vi "Main (RT).vi"() -> ()   [LabVIEW 2015]
uses:
  BMP085 (GY-65) Library/BMP085 (RT).lvlib
panel:
  out "History":cluster{"Temp [°C]":dbl, "hPa":dbl}(graph)
  in  "Stop Button":bool
  out "Pressure [hPa]":dbl(knob) scale=900.0..1100.0
  out "Temperature [°C]":dbl(slide) scale=0.0..80.0
  # "952"
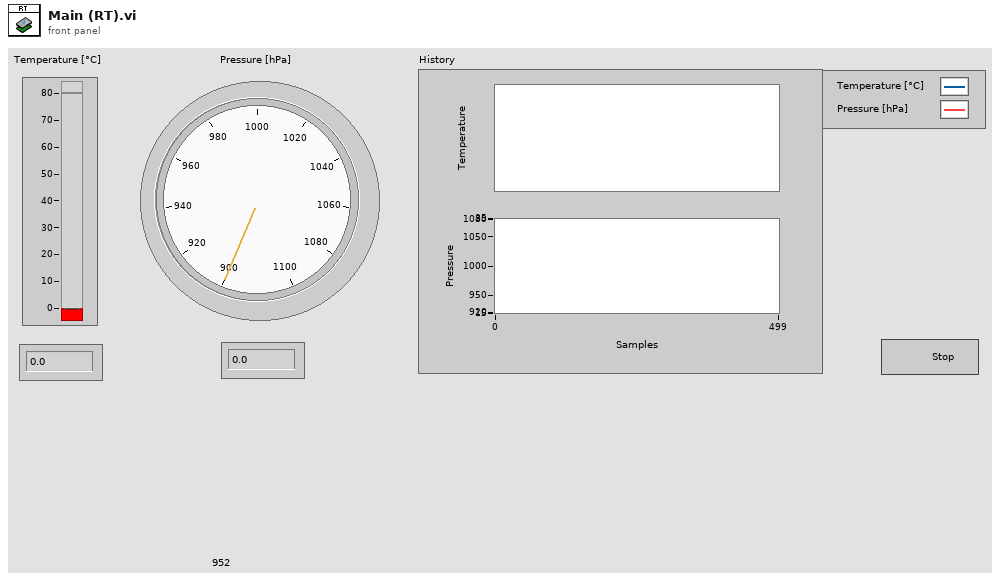
[diagram p1: front panel]
types:
  T1 = enum8{"ultra low power", "standard", "high resolution", "ultra high resolution"}
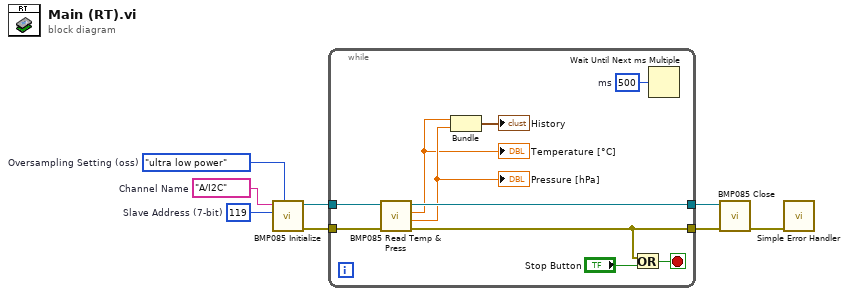
[diagram p0: block diagram]
diagram:
  w3 = u8 119  # Slave Address (7-bit)
  w4 = T1."ultra low power"  # Oversampling Setting (oss)
  w5 = tag "A/I2C"  # Channel Name
  n1 = call "BMP085 Initialize.vi"("Oversampling Setting (oss)"=w4, "Slave Address (7-bit)"=w3, "Channel Name"=w5) -> ("error out"=w7:errorcluster, "BMP085 (GY-65) out"=w8:refnum<class "BMP085 (GY-65).lvclass">)  [unwired: 7 in]
  n2 = while {
    tunnel: w8 -> [w18]
    tunnel: [w17] -> w1
    tunnel: w7 -> [w16]
    tunnel: [w14] -> w6
    stop <- w15 stop-if-true
    w12 = u32 500  # ms
    # "Example: BMP085"
    n3 = call "BMP085 Read Temp & Press.vi"("error in (no error)"=w16, "BMP085 (GY-65) in"=w18) -> ("error out"=w14:errorcluster, "hPa"=w11:dbl, "Temp [°C]"=w10:dbl, "BMP085 (GY-65) out"=w17:refnum<class "BMP085 (GY-65).lvclass">)  [unwired: 6 in]
    "Pressure [hPa]" <- w11
    "Temperature [°C]" <- w10
    n4 = Bundle("Temp [°C]"=w10, "hPa"=w11) -> (→"History":cluster{"Temp [°C]":dbl, "hPa":dbl})  [unwired: 1 in]
    n5 = Or(x=w14, y="Stop Button") -> (x .or. y?=w15:bool)
    n6 = Wait Until Next ms Multiple(millisecond multiple=w12) -> ()  [unwired: 1 out]
  }
  n7 = call "BMP085 Close.vi"("error in (no error)"=w6, "BMP085 (GY-65) in"=w1) -> ("error out"=w2:errorcluster)  [unwired: 9 in]
  n8 = call <vilib>:"Simple Error Handler.vi"("error in (no error)"=w2) -> ()  [unwired: 4 in, 5 out]
